vi "SVR_debug.vi"(8 "error in (no error)":errorcluster, 11 "Gserver in":refnum<class "Gserver.lvclass">) -> (0 "error out":errorcluster, 3 "Gserver out":refnum<class "Gserver.lvclass">)   [LabVIEW 2020, in "Sgraph_lib_V1.lvlib" / "Gserver.lvclass"]
doc: "Andre Koelewijn, 20 July 2021\n\nDebug functions. Should not be active in normal operation"
uses:
  Gserver.lvclass
  Gserver.lvclass/Gserver.ctl
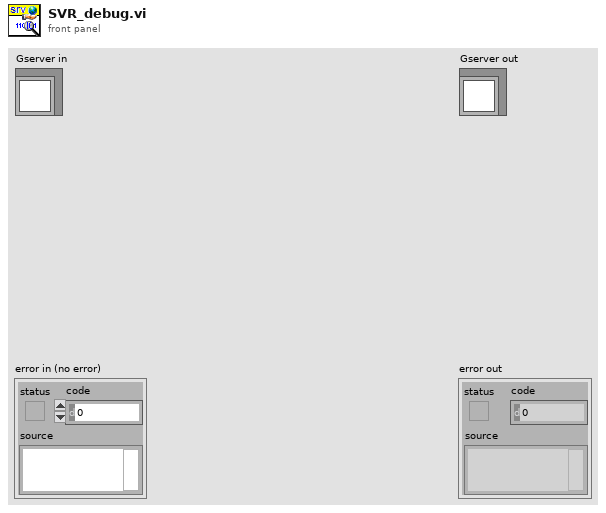
[diagram p1: front panel]
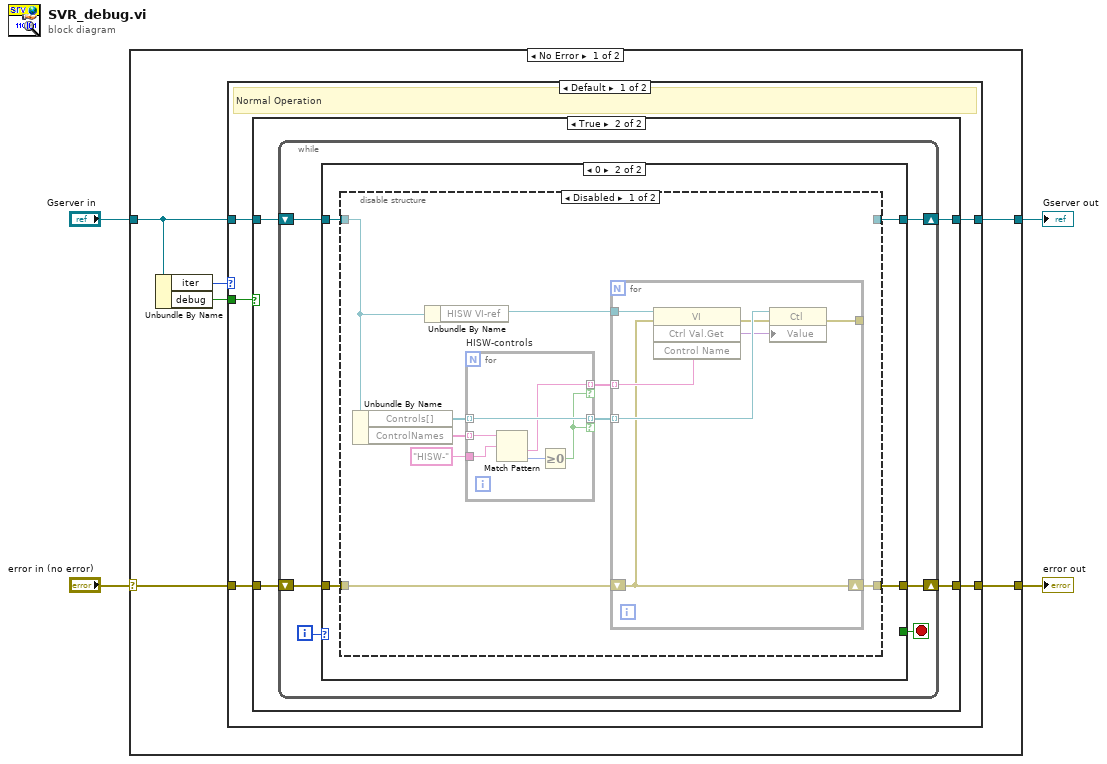
[diagram p0: block diagram]
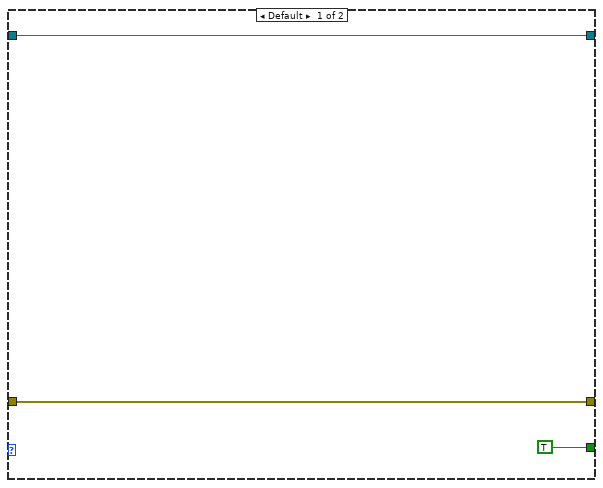
[diagram p3: hidden frame]
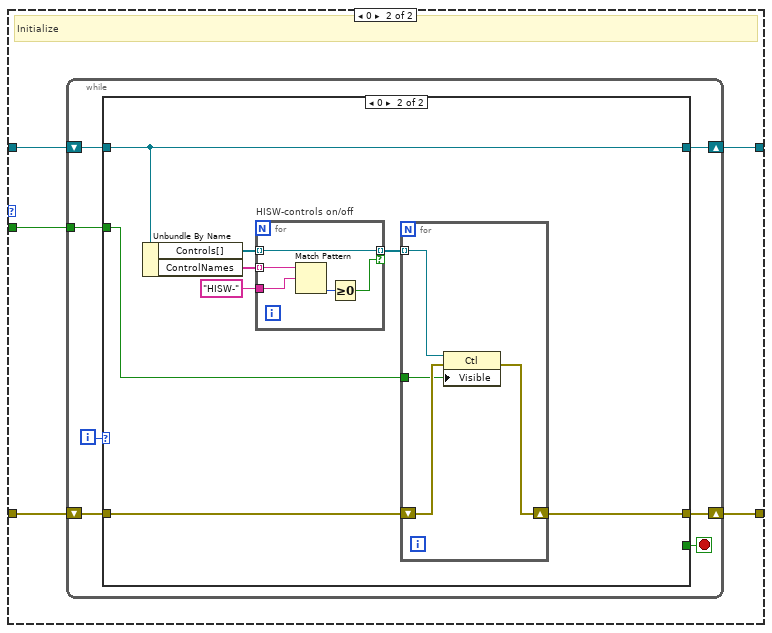
[diagram p5: hidden frame]
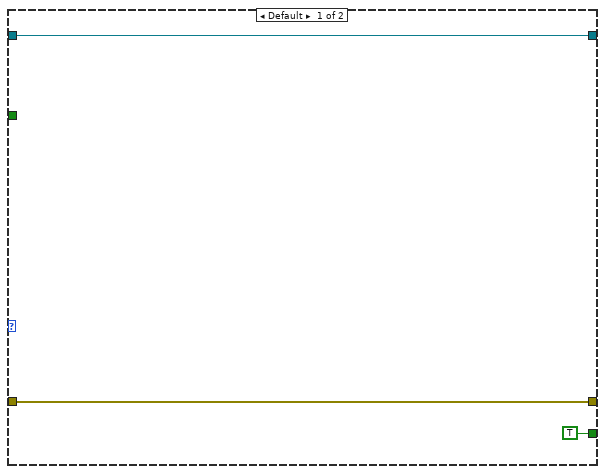
[diagram p6: hidden frame]
diagram:
  n1 = case shown="No Error" "error in (no error)" {
    selector: "error in (no error)" -> [w8 w92]
    tunnel: [w7 w92] -> w3
    tunnel: [w6 w91] -> w1
    tunnel: "Gserver in" -> [w9 w91]
    frame No Error {
      n2 = Unbundle By Name(w9) -> ("iter"=w10:u64, "debug"=w5:bool)
      n3 = case shown="Default" w10 {
        tunnel: w9 -> [w14 w62]
        tunnel: w8 -> [w13 w63]
        tunnel: [w12 w60] -> w7
        tunnel: [w11 w61] -> w6
        tunnel: w5 -> [w15 w59]
        frame Default {
          # "Normal Operation"
          n4 = case shown="True" w15 {
            tunnel: w14 -> [w16 w21]
            tunnel: w13 -> [w17 w20]
            tunnel: [w17 w18] -> w12
            tunnel: [w16 w19] -> w11
            frame False {
            }
            frame True {
              n5 = while {
                shift-right: [w25] -> w19
                shift-left: w21 -> [w26]
                shift-right: [w23] -> w18
                shift-left: w20 -> [w24]
                i -> [w27]
                stop <- w22 stop-if-true
                n6 = case shown="0" w27 {
                  tunnel: w26 -> [w30 w34]
                  tunnel: [w30 w31] -> w25
                  tunnel: w24 -> [w29 w33]
                  tunnel: [w29 w32] -> w23
                  tunnel: [TRUE _] -> w22
                  frame Default {
                  }
                  frame 0 {
                    n7 = disable-structure shown="Disabled" {
                      disable-tunnel: w34 -> [w40 w58]
                      disable-tunnel: w33 -> [w36 w57]
                      disable-tunnel: [w35 w57] -> w32
                      disable-tunnel: [_ w58] -> w31
                      frame Disabled {
                        n8 = Unbundle By Name(w40) -> ("Controls[]"=w41:refnum<vi>[], "ControlNames"=w43:string[])
                        n9 = Unbundle By Name(w40) -> ("HISW VI-ref"=w39:refnum<vi>)
                        n10 = for "HISW-controls" {
                          tunnel: w43 -> [w53] mode=indexing
                          tunnel: "HISW-" -> [w56]
                          tunnel: w41 -> [w55] mode=indexing
                          tunnel: [w55] -> w37 mode=indexing if=w52
                          tunnel: [w51] -> w38 mode=indexing if=w52
                          n11 = Match Pattern(string=w53, regular expression=w56) -> (after substring=w51:string, offset past match=w54:i32)  [unwired: 1 in, 2 out]
                          n12 = Greater Or Equal To 0?(x=w54) -> (x >= 0?=w52:bool)
                        }
                        n13 = for {
                          tunnel: w39 -> [w50]
                          tunnel: w38 -> [w49] mode=indexing
                          tunnel: w37 -> [w48] mode=indexing
                          shift-right: [w45] -> w35
                          shift-left: w36 -> [w45]
                          tunnel: [w44] -> _
                          n14 = invoke class="VI" method="Ctrl Val.Get"(reference=w50, error in=w45, "Control Name"=w49) -> (error out=w46:errorcluster, "Get Control Value Variant"=w47:variant)  [unwired: 1 in, 2 out]
                          n15 = property class="Ctl"(reference=w48, error in=w46, "Value"=w47) -> (error out=w44:errorcluster)  [unwired: 1 out]
                        }
                      }
                      frame Enabled {
                      }
                    }
                  }
                }
              }
            }
          }
        }
        frame 0 {
          # "Initialize"
          n16 = while {
            shift-right: [w66] -> w61
            shift-left: w62 -> [w67]
            shift-right: [w68] -> w60
            shift-left: w63 -> [w69]
            tunnel: w59 -> [w64]
            i -> [w70]
            stop <- w65 stop-if-true
            n17 = case shown="0" w70 {
              tunnel: w69 -> [w72 w76]
              tunnel: [w72 w75] -> w68
              tunnel: w67 -> [w73 w79]
              tunnel: [w73 w79] -> w66
              tunnel: [TRUE _] -> w65
              tunnel: w64 -> [_ w74]
              frame Default {
              }
              frame 0 {
                n18 = Unbundle By Name(w79) -> ("Controls[]"=w78:refnum<vi>[], "ControlNames"=w81:string[])
                n19 = for "HISW-controls on/off" {
                  tunnel: w81 -> [w90] mode=indexing
                  tunnel: "HISW-" -> [w89]
                  tunnel: w78 -> [w88] mode=indexing
                  tunnel: [w88] -> w77 mode=indexing if=w86
                  n20 = Match Pattern(string=w90, regular expression=w89) -> (offset past match=w87:i32)  [unwired: 1 in, 3 out]
                  n21 = Greater Or Equal To 0?(x=w87) -> (x >= 0?=w86:bool)
                }
                n22 = for {
                  tunnel: w77 -> [w85] mode=indexing
                  shift-right: [w83] -> w75
                  shift-left: w76 -> [w84]
                  tunnel: w74 -> [w82]
                  n23 = property class="Ctl"(reference=w85, error in=w84, "Visible"=w82) -> (error out=w83:errorcluster)  [unwired: 1 out]
                }
              }
            }
          }
        }
      }
    }
    frame Error {
    }
  }
  "error out" <- w3
  "Gserver out" <- w1
